vi "Main.vi"() -> ()   [LabVIEW 2022 SP3]
uses:
  Consumer Message.ctl
  <vilib>/Utility/error.llb/Error Cluster From Error Code.vi
  <vilib>/ErrorRing/Error Ring.xnode
panel:
  in  "Producer Error":bool
  in  "Consumer Error":bool
  out "Consumer Shutdown?":bool
  out "State to Execute":string
  out "High Priority?":bool
  out "Backlog":u8(slide) scale=0.0..100.0
  out "Processed Value":i32
  in  "High Priority Message":bool
  in  "Normal Priority Message":bool
  in  "Stop":bool
  # "Number of enqueued\nmessages waiting to\nbe processed"
  # "Current data being\nprocessed in consumer loop"
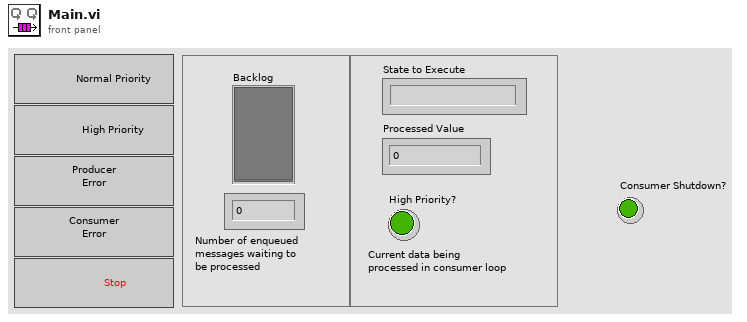
[diagram p1: front panel]
types:
  T1 = typedef "Consumer Message.ctl" = cluster{"Consumer State":string, "Boolean Data":bool, "Numeric Data":i32, "Error":errorcluster}
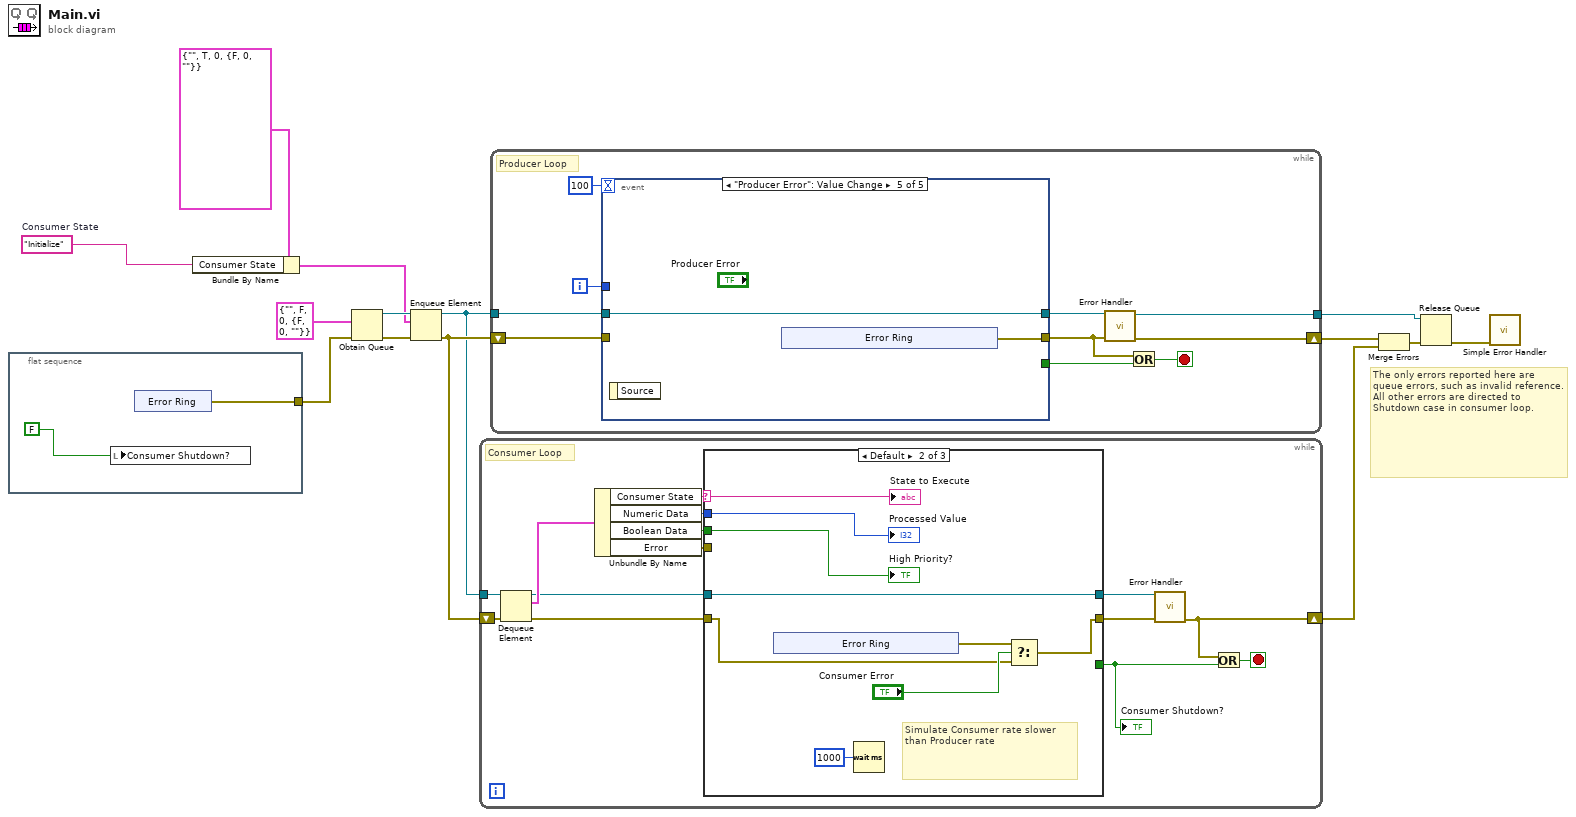
[diagram p0: block diagram]
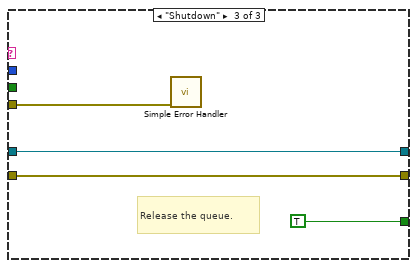
[diagram p3: hidden frame]
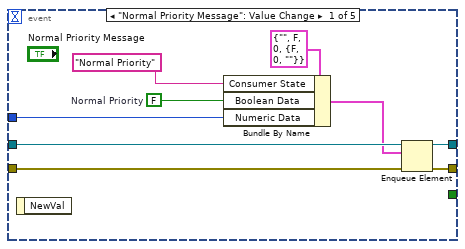
[diagram p4: hidden frame]
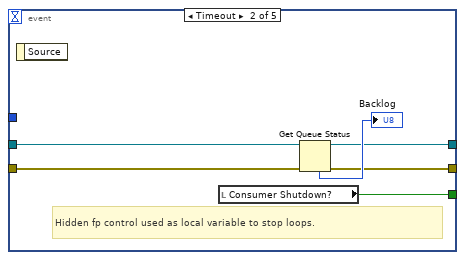
[diagram p5: hidden frame]
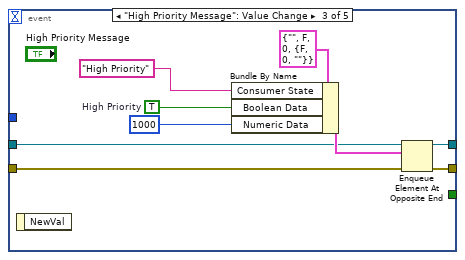
[diagram p6: hidden frame]
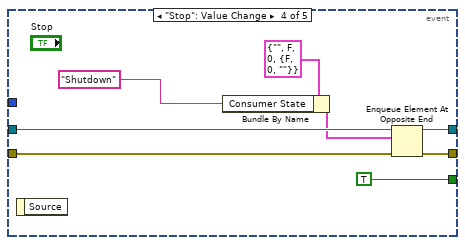
[diagram p7: hidden frame]
diagram:
  w6 = "Initialize"  # Consumer State
  # "The only errors reported here are queue errors, such as invalid reference.  All other errors are directed to Shutdown case in consumer loop."
  n1 = flat-sequence {
    tunnel: [w15] -> w9
    frame #0 {
      n2 = local write "Consumer Shutdown?"(FALSE ("Stop Loops (local)")) -> ()
      n3 = xnode "Error Ring"() -> ("error out"=w15:errorcluster)
    }
  }
  n4 = Bundle By Name(cluster=T1 {"Consumer State"="", "Boolean Data"=TRUE, "Numeric Data"=0, "Error"={"status"=FALSE, "code"=0, "source"=""}} ("Consumer Message"), "Consumer State"=w6) -> (w7:T1)
  n5 = Obtain Queue(element data type=T1 {"Consumer State"="", "Boolean Data"=FALSE, "Numeric Data"=0, "Error"={"status"=FALSE, "code"=0, "source"=""}}, error in (no error)=w9) -> (queue out=w11:refnum<queue>, error out=w14:errorcluster)  [unwired: 3 in, 1 out]
  n6 = Enqueue Element(queue=w11, element=w7, error in (no error)=w14) -> (queue out=w10:refnum<queue>, error out=w12:errorcluster)  [unwired: 1 in, 1 out]
  n7 = while {
    tunnel: w10 -> [w31]
    shift-right: [w20] -> w5
    shift-left: w12 -> [w30]
    stop <- w21 stop-if-true
    # "Consumer Loop"
    n8 = Dequeue Element(queue=w31, error in (no error)=w30) -> (queue out=w19:refnum<queue>, element=w29:T1, error out=w18:errorcluster)  [unwired: 1 in, 1 out]
    n9 = Unbundle By Name(w29) -> ("Consumer State"=w28:string, "Numeric Data"=w27:i32, "Boolean Data"=w26:bool, "Error"=w23:errorcluster)
    n10 = case shown="Default" w28 {
      selector: w28 -> [_ w39 _]
      tunnel: [_ _ TRUE] -> w22
      tunnel: w18 -> [w32 w35 w48]
      tunnel: [w32 w34 w48] -> w25
      tunnel: w27 -> [_ w42 _]
      tunnel: w26 -> [_ w41 _]
      tunnel: w19 -> [w33 w40 w49]
      tunnel: [w33 w40 w49] -> w24
      tunnel: w23 -> [_ _ w50]
      frame "Initialize" {
      }
      frame Default {
        # "Simulate Consumer rate slower than Producer rate"
        n11 = xnode "Error Ring"() -> ("error out"=w37:errorcluster)
        n12 = Wait (ms)(milliseconds to wait=u32 1000) -> ()  [unwired: 1 out]
        n13 = Select(t=w37, s="Consumer Error", f=w35) -> (s? t:f=w34:errorcluster)
        "Processed Value" <- w42
        "High Priority?" <- w41
        "State to Execute" <- w39
      }
      frame "Shutdown" {
        # "Release the queue."
        n14 = call <vilib>:"Simple Error Handler.vi"("error in (no error)"=w50) -> ()  [unwired: 4 in, 5 out]
      }
    }
    "Consumer Shutdown?" <- w22
    n15 = call "Error Handler.vi"("error in"=w25, "queue in"=w24) -> ("error out"=w20:errorcluster)  [unwired: 8 in, 1 out]
    n16 = Or(x=w20, y=w22) -> (x .or. y?=w21:bool)
  }
  n17 = while {
    tunnel: w10 -> [w61]
    shift-right: [w53] -> w4
    shift-left: w12 -> [w60]
    tunnel: [w52] -> w1
    i -> [w59]
    stop <- w55 stop-if-true
    # "Producer Loop"
    n18 = event shown="[4] \"Producer Error\": Value Change" {
      selector: _ -> [_ _ _ _ _]
      dyn-events: _ -> [_ _ _ _ _]
      timeout: 100 -> [_ _ _ _ _]
      tunnel: w61 -> [w70 w74 w77 w93 w95]
      tunnel: w60 -> [w68 w73 w84 w91 _]
      tunnel: [w69 w72 w85 w90 w94] -> w54
      tunnel: [_ w76 _ TRUE _] -> w56
      tunnel: w59 -> [w67 _ _ _ _]
      tunnel: [w63 w71 w80 w89 w95] -> w58
      event "Normal Priority Message": Value Change {
        w64 = FALSE  # Normal Priority
        n19 = event-data() -> ()  [unwired: 1 in, 1 out]
        n20 = Bundle By Name(cluster=T1 {"Consumer State"="", "Boolean Data"=FALSE, "Numeric Data"=0, "Error"={"status"=FALSE, "code"=0, "source"=""}}, "Consumer State"="Normal Priority" ("String Data"), "Boolean Data"=w64, "Numeric Data"=w67) -> (w66:T1)
        n21 = Enqueue Element(queue=w70, element=w66, error in (no error)=w68) -> (queue out=w63:refnum<queue>, error out=w69:errorcluster)  [unwired: 1 in, 1 out]
      }
      event Timeout {
        # "Hidden fp control used as local variable to stop loops."
        n22 = event-data() -> ()  [unwired: 1 in, 1 out]
        n23 = local read "Consumer Shutdown?"() -> (w76:bool)
        n24 = Get Queue Status(queue=w74, error in (no error)=w73) -> (queue out=w71:refnum<queue>, error out=w72:errorcluster, # elements in queue=→"Backlog":i32)  [unwired: 1 in, 5 out]
      }
      event "High Priority Message": Value Change {
        w79 = TRUE  # High Priority
        n25 = event-data() -> ()  [unwired: 1 in, 1 out]
        n26 = Bundle By Name(cluster=T1 {"Consumer State"="", "Boolean Data"=FALSE, "Numeric Data"=0, "Error"={"status"=FALSE, "code"=0, "source"=""}}, "Consumer State"="High Priority" ("String Data"), "Boolean Data"=w79, "Numeric Data"=1000) -> (w82:T1)
        n27 = Enqueue Element At Opposite End(queue=w77, element=w82, error in (no error)=w84) -> (queue out=w80:refnum<queue>, error out=w85:errorcluster)  [unwired: 1 in, 1 out]
      }
      event "Stop": Value Change {
        n28 = event-data() -> ()  [unwired: 1 in, 1 out]
        n29 = Bundle By Name(cluster=T1 {"Consumer State"="", "Boolean Data"=FALSE, "Numeric Data"=0, "Error"={"status"=FALSE, "code"=0, "source"=""}}, "Consumer State"="Shutdown") -> (w86:T1)
        n30 = Enqueue Element At Opposite End(queue=w93, element=w86, error in (no error)=w91) -> (queue out=w89:refnum<queue>, error out=w90:errorcluster)  [unwired: 1 in, 1 out]
      }
      event "Producer Error": Value Change {
        n31 = event-data() -> ()  [unwired: 1 in, 1 out]
        n32 = xnode "Error Ring"() -> ("error out"=w94:errorcluster)
      }
    }
    n33 = call "Error Handler.vi"("error in"=w54, "queue in"=w58) -> ("error out"=w53:errorcluster, "queue out"=w52:refnum<queue>)  [unwired: 8 in]
    n34 = Or(x=w54, y=w56) -> (x .or. y?=w55:bool)
  }
  n35 = Merge Errors(w4, w5) -> (w3:errorcluster)
  n36 = Release Queue(queue=w1, error in (no error)=w3) -> (error out=w2:errorcluster)  [unwired: 1 in, 2 out]
  n37 = call <vilib>:"Simple Error Handler.vi"("error in (no error)"=w2) -> ()  [unwired: 4 in, 5 out]
